vi "ADXL345 I2C Read.vi"(8 "error in":errorcluster, 10 "Axis":T3 items=["X-Axis", "Y-Axis", "Z-Axis"], 11 "I2CDevRef":T1 {"Device Address" format="%.0x"}) -> (0 "error out":errorcluster, 2 "Acceleration":dbl, 3 "I2CDevRef Out":T1 {"Device Address" format="%.0x"})   [LabVIEW 2012]
uses:
  ADXL345 I2C Axis.ctl
  <vilib>/Rock Robotics/WPI/I2C/WPI_I2CDevRef.ctl
  <vilib>/Rock Robotics/SystemInterfaces/Typedef/FPGA_TypedefDigitalModule.ctl
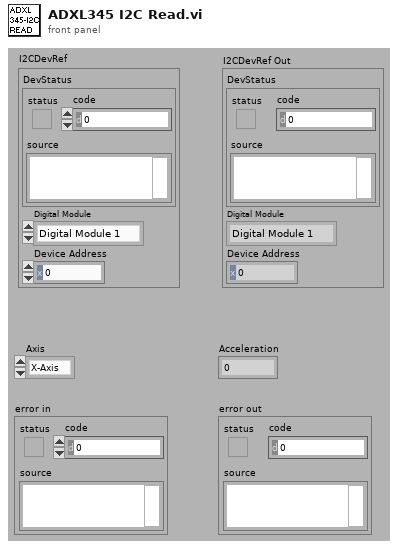
[diagram p1: front panel]
types:
  T1 = typedef "WPI_I2CDevRef.ctl" = cluster{"DevStatus":errorcluster, "Digital Module":T2, "Device Address":u8}
  T2 = typedef "FPGA_TypedefDigitalModule.ctl" = enum16{"Digital Module 1", "Digital Module 2"}
  T3 = typedef "ADXL345 I2C Axis.ctl" = u8
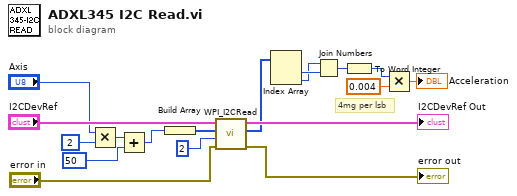
[diagram p0: block diagram]
diagram:
  # "4mg per lsb"
  n1 = Multiply(x="Axis", y=u8 2 ("Data To Send")) -> (x*y=w18:T3)
  n2 = Add(x=w18, y=u8 50 ("Data To Send")) -> (x+y=w5:T3)
  n3 = Build Array(w5) -> (w4:T3[])
  n4 = call <vilib>:"WPI_I2CRead.vi"("error in (no error)"="error in", "I2CBytesToRead"=u8 2, "I2CRegister"=w4, "I2CDevRef"="I2CDevRef") -> ("error out"=→"error out":errorcluster, "Data Out"=w9:u8[], "I2CDevRef"=→"I2CDevRef Out":T1)  [unwired: 1 in, 4 out]
  n5 = Index Array(array=w9) -> (element #1=w7:u8, element #2=w6:u8)  [unwired: 2 in]
  n6 = Join Numbers(hi=w6, lo=w7) -> ((hi.lo)=w8:u16)
  n7 = To Word Integer(number=w8) -> (16bit integer=w1:i16)
  n8 = Multiply(x=w1, y=0.004) -> (x*y=→"Acceleration":dbl)
